vi "CALC_MARK_DISC_ON_OFF.vi"(0 "VISA IN":refnum<visa-resource-name>, 1 "Marker number":i32, 2 "Actual(ON) or Calculated(OFF) Data":bool, 5 "error in":errorcluster, 7 "Channel":i32) -> (14 "VISA Out":refnum<visa-resource-name>, 19 "error out":errorcluster)   [LabVIEW 2018, in "PNA-X.lvlib"]
doc: "CALCulate<cnum>:MARKer<mkr>:DISCrete <ON|OFF> \n(Read-Write) Makes the specified marker display either a calculated value between data points \n(interpolated data) or the actual data points (discrete data). \nSee Critical Note \nParameters \n<cnum> Channel number of the measurement. There must be a selected measurement \non that channel. If unspecified, <cnum> is set to 1. \n<mkr> Any existing marker number from 1 to 10; if unspecified, value is set to 1. \n<ON|OFF> ON (or 1) - Specified marker displays the actual data points \nOFF (or 0) - Specified marker displays calculated data between the actual data \npoints. \nExamples CALC:MARK:DISC ON \ncalculate2:marker8:discrete off \nQuery Syntax CALCulate<cnum>:MARKer<mkr>:DISCrete? \nReturn Type Boolean (1 = ON, 0 = OFF) \nDefault OFF \n1530"
uses:
  PNA-X.lvlib
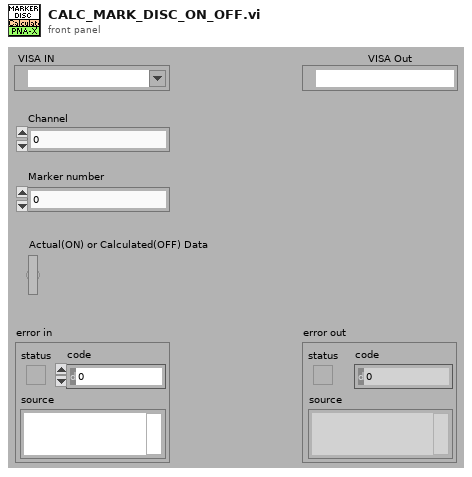
[diagram p1: front panel]
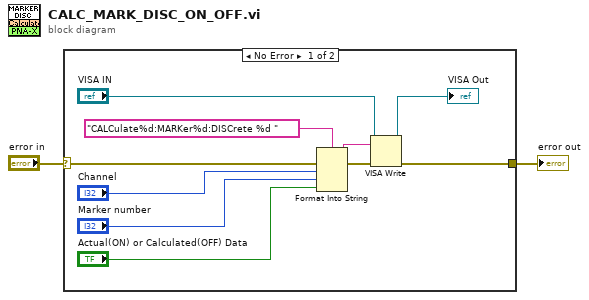
[diagram p0: block diagram]
diagram:
  n1 = case shown="No Error" "error in" {
    selector: "error in" -> [w12 w13]
    tunnel: [w7 w13] -> w1
    frame No Error {
      n2 = Format Into String(format string="CALCulate%d:MARKer%d:DISCrete %d " ("Cmdline"), error in=w12, "Channel", "Marker number", "Actual(ON) or Calculated(OFF) Data") -> (resulting string=w10:string, error out=w11:errorcluster)  [unwired: 1 in]
      n3 = VISA Write(VISA resource name="VISA IN", write buffer=w10, error in (no error)=w11) -> (VISA resource name out=→"VISA Out":refnum<visa-resource-name>, error out=w7:errorcluster)  [unwired: 1 out]
    }
    frame Error {
    }
  }
  "error out" <- w1
